vi "Recalculate Stats.vi"(9 "Dump Stat":T2, 10 "Levels Available":i32, 11 "Levels":T1) -> (2 "Levels Remaining":i32, 3 "Levels out":T1, 5 "Valid?":bool)   [LabVIEW 2023]
uses:
  CTLs/Dump Stat.ctl
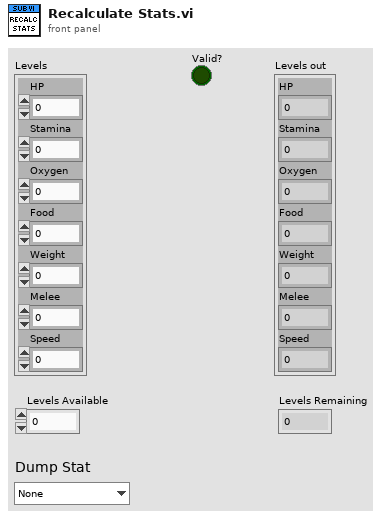
[diagram p1: front panel]
types:
  T1 = cluster{"HP":i32, "Stamina":i32, "Oxygen":i32, "Food":i32, "Weight":i32, "Melee":i32, "Speed":i32}
  T2 = typedef "Dump Stat.ctl" = enum16{"None", "HP", "Stamina", "Oxygen", "Food", "Weight", "Melee", "Speed"}
  T3 = cluster{"Levels[0]":i32, "Levels[1]":i32, "Levels[2]":i32, "Levels[3]":i32, "Levels[4]":i32, "Levels[5]":i32, "Levels[6]":i32}
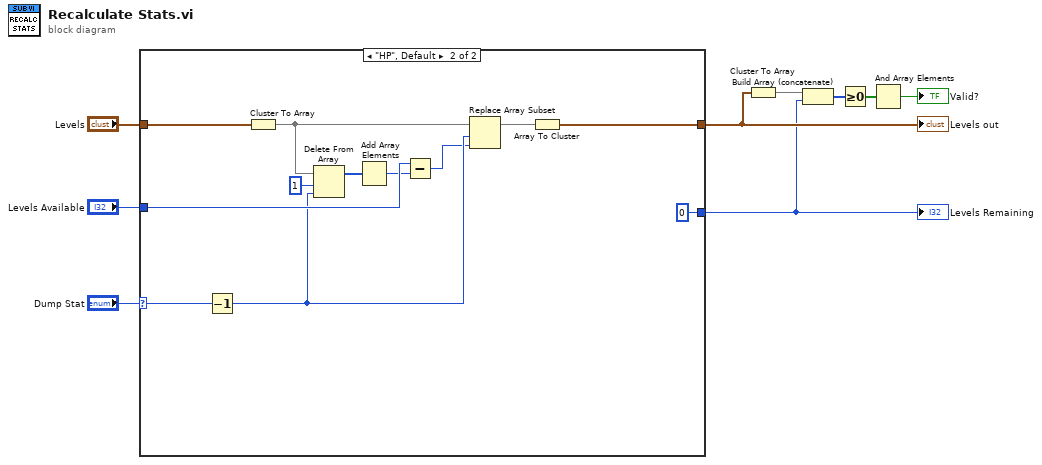
[diagram p0: block diagram]
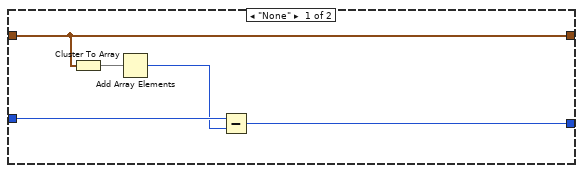
[diagram p2: hidden frame]
diagram:
  n1 = case shown="\"HP\", Default" "Dump Stat" {
    selector: "Dump Stat" -> [_ w24]
    tunnel: "Levels" -> [w14 w25]
    tunnel: "Levels Available" -> [w12 w21]
    tunnel: [w14 w15] -> w6
    tunnel: [w10 0] -> w3
    frame "None" {
      n2 = Cluster To Array(cluster=w14) -> (array=w13:i32[])
      n3 = Add Array Elements(numeric array=w13) -> (sum=w11:i32)
      n4 = Subtract(x=w12, y=w11) -> (x-y=w10:i32)
    }
    frame "HP", Default {
      n5 = Decrement(x=w24) -> (x-1=w18:T2)
      n6 = Cluster To Array(cluster=w25) -> (array=w19:i32[])
      n7 = Delete From Array(array=w19, length=1, index=w18) -> (array with subset deleted=w22:i32[])  [unwired: 1 out]
      n8 = Add Array Elements(numeric array=w22) -> (sum=w20:i32)
      n9 = Subtract(x=w21, y=w20) -> (x-y=w17:i32)
      n10 = Replace Array Subset(array=w19, new element=w17, index=w18) -> (w16:i32[])
      n11 = Array To Cluster(array=w16) -> (cluster=w15:T3)
    }
  }
  "Levels Remaining" <- w3
  "Levels out" <- w6
  n12 = Cluster To Array(cluster=w6) -> (array=w4:i32[])
  n13 = Build Array (concatenate)(w4, w3) -> (w2:i32[])
  n14 = Greater Or Equal To 0?(x=w2) -> (x >= 0?=w5:bool[])
  n15 = And Array Elements(Boolean array=w5) -> (logical AND=→"Valid?":bool)
